vi "Set Voltage and Current.vi"(6 "channel (1)":u8=1 min=1 max=4 step=1, 8 "error in (no error)":errorcluster, 9 "current (0 A)":dbl=0.13 format="%.3f", 10 "voltage (0 V)":dbl format="%.3f", 11 "VISA resource name":refnum<visa-resource-name>) -> (0 "error out":errorcluster, 3 "VISA resource name out":refnum<visa-resource-name>)   [LabVIEW 2020, in "Agilent 6XXX Series.lvlib"]
doc: "This function sets the voltage (in Volts) and current (in Amps) of the instrument."
uses:
  <instrlib>/Agilent 6XXX Series/Agilent 6XXX Series.lvlib
panel:
  # "*662xA only"
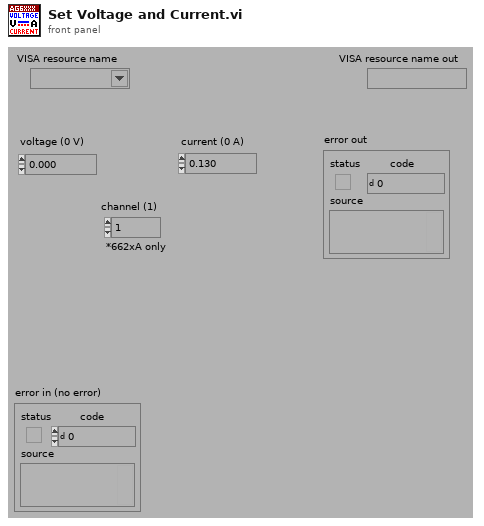
[diagram p1: front panel]
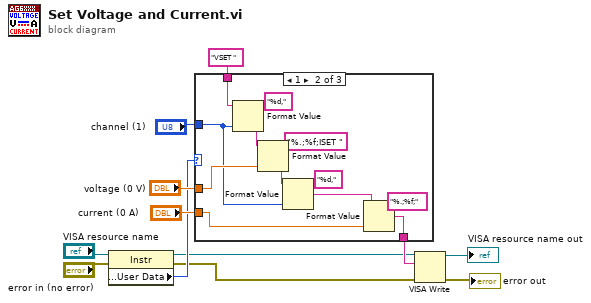
[diagram p0: block diagram]
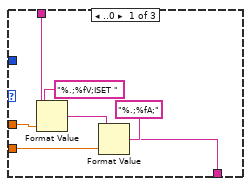
[diagram p2: hidden frame]
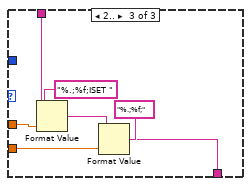
[diagram p3: hidden frame]
diagram:
  n1 = property class="Instr"(reference="VISA resource name", error in="error in (no error)") -> (reference out=w3:refnum<visa-resource-name>, error out=w2:errorcluster, "General Settings:User Data"=w4:u32)
  n2 = case shown="1" w4 {
    tunnel: "VSET " -> [w18 w28 w37]
    tunnel: [w13 w30 w32] -> w12
    tunnel: "voltage (0 V)" -> [w15 w22 w34]
    tunnel: "current (0 A)" -> [w14 w21 w33]
    tunnel: "channel (1)" -> [_ w20 _]
    frame ..0 {
      n3 = Format Value(string ("")=w18, format string="%.;%fV;ISET ", value (0)=w15) -> (output string=w17:string)
      n4 = Format Value(string ("")=w17, format string="%.;%fA;", value (0)=w14) -> (output string=w13:string)
    }
    frame 1 {
      n5 = Format Value(string ("")=w28, format string="%d,", value (0)=w20) -> (output string=w26:string)
      n6 = Format Value(string ("")=w26, format string="%.;%f;ISET ", value (0)=w22) -> (output string=w23:string)
      n7 = Format Value(string ("")=w23, format string="%d,", value (0)=w20) -> (output string=w24:string)
      n8 = Format Value(string ("")=w24, format string="%.;%f;", value (0)=w21) -> (output string=w30:string)
    }
    frame 2.. {
      n9 = Format Value(string ("")=w37, format string="%.;%f;ISET ", value (0)=w34) -> (output string=w36:string)
      n10 = Format Value(string ("")=w36, format string="%.;%f;", value (0)=w33) -> (output string=w32:string)
    }
  }
  n11 = VISA Write(VISA resource name=w3, write buffer=w12, error in (no error)=w2) -> (VISA resource name out=→"VISA resource name out":refnum<visa-resource-name>, error out=→"error out":errorcluster)  [unwired: 1 out]
